vi "send engine statuses.vi"(8 "error in":errorcluster, 10 "statuses":T1[](array[typedef]), 11 "message queue in":T5) -> (0 "error out":errorcluster, 3 "message queue out":T5)   [LabVIEW 2013, in "DCAF message service.lvlib"]
uses:
  DCAF message service.lvlib
  <vilib>/NI/AMC/Message Queue.ctl
  <vilib>/NI/AMC/Message.ctl
  <vilib>/NI/Tools/Keyed Array/KeyedArray.ctl
  engine status data.ctl
  <vilib>/NI/Module Execution Interface/Engine Runtime/Execution States.ctl
  <vilib>/NI/Module Execution Interface/Engine Runtime/Fault.ctl
  <vilib>/NI/Tag Bus Module Framework/runtime/error classification.ctl
  common reponses to network process.ctl
  <vilib>/NI/AMC/Create Single Message.vi
  <vilib>/NI/AMC/Update Message Routing Info.vi
  <vilib>/NI/AMC/Send Message.vi
  <vilib>/NI/AMC/AMC.lvlib
  <vilib>/NI/Tools/Keyed Array/Tools_KeyedArray.lvlib
  <vilib>/NI/Module Execution Interface/Engine Runtime/Engine Runtime Interface.lvclass
  <vilib>/NI/Tag Bus Module Framework/runtime/TBM module execution interface.lvclass
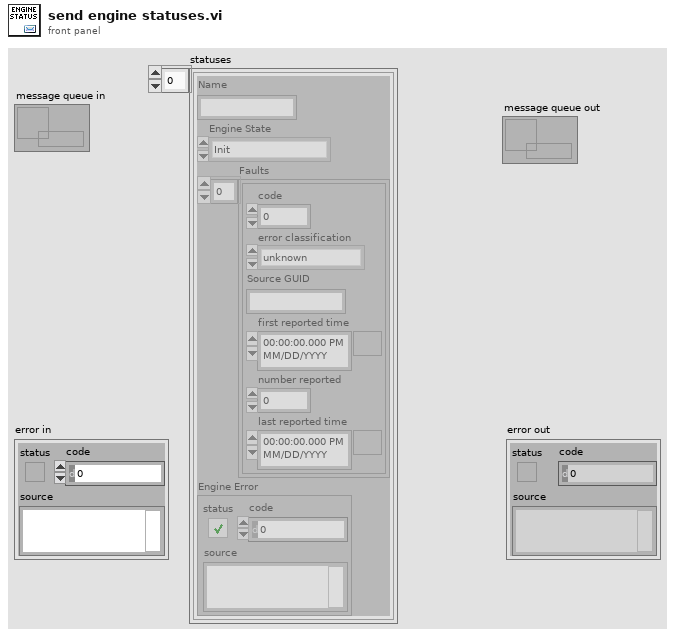
[diagram p1: front panel]
types:
  T1 = typedef "DCAF message service.lvlib/engine status data.ctl" = cluster{"Name":string, "Engine State":T2, "Faults":T3[], "Engine Error":errorcluster}
  T2 = typedef "Engine Runtime Interface.lvclass/Execution States.ctl" = enum16{"Init", "Pre-Operational", "Safe-Operational", "Operational", "Stopped"}
  T3 = typedef "Engine Runtime Interface.lvclass/Fault.ctl" = cluster{"code":i32, "error classification":T4, "Source GUID":string, "first reported time":timestamp, "number reported":u32, "last reported time":timestamp}
  T4 = typedef "TBM module execution interface.lvclass/error classification.ctl" = enum16{"unknown", "none", "trivial", "recoverable", "critical"}
  T5 = typedef "AMC.lvlib/Message Queue.ctl" = refnum<queue>
  T6 = typedef "DCAF message service.lvlib/common reponses to network process.ctl" = enum16{"System Error", "Load Report", "Action Response", "Engine Status"}
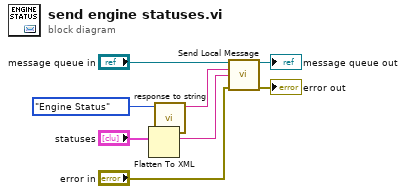
[diagram p0: block diagram]
diagram:
  n1 = Flatten To XML(anything="statuses") -> (xml string=w5:string)
  n2 = call "response to string.vi"("responses"=common_reponses_to_network_process."Engine Status") -> ("command string"=w2:string)  [unwired: 10 in]
  n3 = call <vilib>:"Send Local Message.vi"("message queue in"="message queue in", "message name"=w2, "message value"=w5, "error in"="error in") -> ("message queue out"=→"message queue out":T5, "error out"=→"error out":errorcluster)  [unwired: 9 in, 1 out]
